vi "DSF.Shared.Configuration.Plugin.Create.vi"(7 "Custom Parameters":variant, 8 "error in (no error)":errorcluster, 9 "Cycle Timing Factors":T1={"Decimation"=1, "Offset"=0}, 10 "Name":string) -> (0 "error out":errorcluster, 3 "Plugin Configuration out":refnum<class "DSF.Shared.Configuration.Plugin.lvclass">)   [LabVIEW 2016, in "DSF.Shared.lvlib" / "DSF.Shared.Configuration.Plugin.lvclass"]
uses:
  DSF.Shared.Configuration.Plugin.lvclass
  Typedefs/DSF.Shared.Typedefs.Cycle Timing Factors.ctl
  DSF.Shared.lvlib
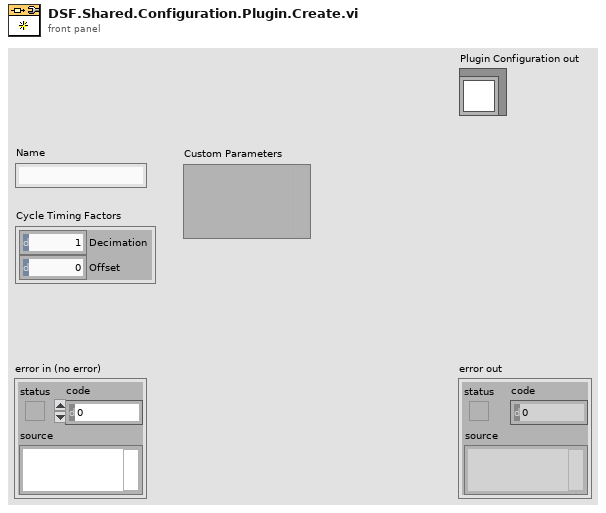
[diagram p1: front panel]
types:
  T1 = typedef "DSF.Shared.lvlib/DSF.Shared.Typedefs.Cycle Timing Factors.ctl" = cluster{"Decimation":u64, "Offset":u64}
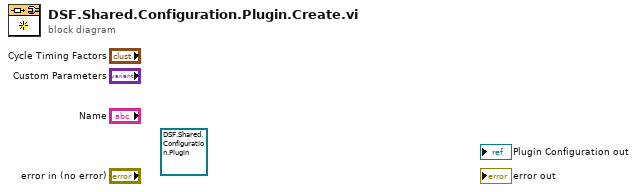
[diagram p0: block diagram]
diagram:
  (unwired) refnum<class "DSF.Shared.Configuration.Plugin.lvclass"> refnum ("Plugin Configuration in")
